vi "mainActivity__关闭所有vi.vi"() -> (0 "所需要关闭的所有vi参数":cluster{"message":string, "data":variant}[](array[cluster]))   [LabVIEW 2014]
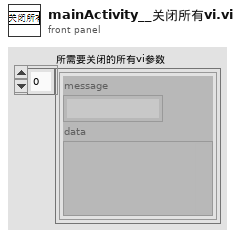
[diagram p1: front panel]
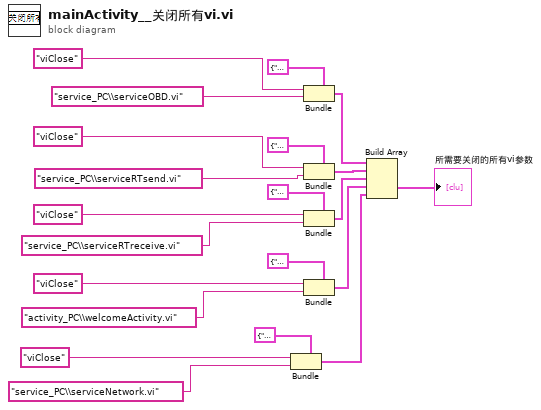
[diagram p0: block diagram]
diagram:
  n1 = Bundle(cluster=cluster{"message":string, "data":variant} {"message"="", "data"=variant} ("元素"), "message"="viClose", "data"="service_PC\\serviceNetwork.vi") -> (w1:cluster{"message":string, "data":variant})
  n2 = Bundle(cluster=cluster{"message":string, "data":variant} {"message"="", "data"=variant} ("元素"), "message"="viClose", "data"="service_PC\\serviceOBD.vi") -> (w14:cluster{"message":string, "data":variant})
  n3 = Bundle(cluster=cluster{"message":string, "data":variant} {"message"="", "data"=variant} ("元素"), "message"="viClose", "data"="service_PC\\serviceRTsend.vi") -> (w15:cluster{"message":string, "data":variant})
  n4 = Bundle(cluster=cluster{"message":string, "data":variant} {"message"="", "data"=variant} ("元素"), "message"="viClose", "data"="service_PC\\serviceRTreceive.vi") -> (w16:cluster{"message":string, "data":variant})
  n5 = Bundle(cluster=cluster{"message":string, "data":variant} {"message"="", "data"=variant} ("元素"), "message"="viClose", "data"="activity_PC\\welcomeActivity.vi") -> (w5:cluster{"message":string, "data":variant})
  n6 = Build Array(w14, w15, w16, w5, w1) -> (→"所需要关闭的所有vi参数":cluster{"message":string, "data":variant}[])
